vi "SIS (SubVI).vi"(8 "SIS-10AI301":dbl, 9 "SIS-10TI101":dbl, 10 "SIS-10LI202":dbl, 11 "SIS-10LI201":dbl) -> (1 "SIS-10SDV501":bool, 2 "SIS-10SDV502":bool, 3 "SIS-10SDV500":bool)   [LabVIEW 2018]
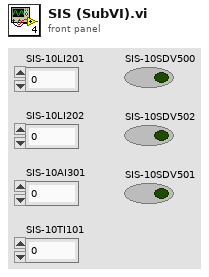
[diagram p1: front panel]
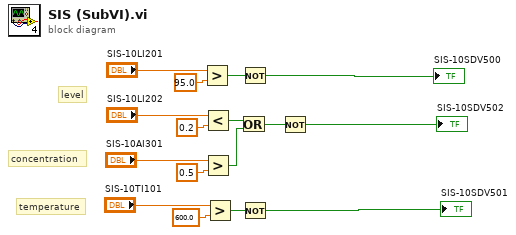
[diagram p0: block diagram]
diagram:
  # "temperature"
  # "concentration"
  # "level"
  n1 = Greater?(x="SIS-10LI201", y=95.0) -> (0:w2:bool)
  n2 = Less?(x="SIS-10LI202", y=0.2) -> (x < y?=w6:bool)
  n3 = Greater?(x="SIS-10AI301", y=0.5) -> (0:w7:bool)
  n4 = Greater?(x="SIS-10TI101", y=600.0) -> (0:w4:bool)
  n5 = Or(x=w6, y=w7) -> (x .or. y?=w8:bool)
  n6 = Not(x=w2) -> (.not. x?=→"SIS-10SDV500":bool)
  n7 = Not(x=w4) -> (.not. x?=→"SIS-10SDV501":bool)
  n8 = Not(x=w8) -> (.not. x?=→"SIS-10SDV502":bool)
